vi "Mathematical interpolation.vi"(10 "Input data":dbl[][](array[numeric]), 11 "Method":i32(ring)=3 items=["nearest", "linear", "spline", "cubic Hermite", "Lagrange"]) -> (2 "Interpolated Data":dbl[][](array[numeric]), 3 "1D Interpolation Graph":cluster{"yi":dbl[], "ramp data":dbl[]}[](graph))   [LabVIEW 2017]
uses:
  <vilib>/Analysis/1siggen.llb/Ramp Pattern by Delta.vi
  <vilib>/gmath/NI_Gmath.lvlib
  <vilib>/Analysis/NI_AALBase.lvlib
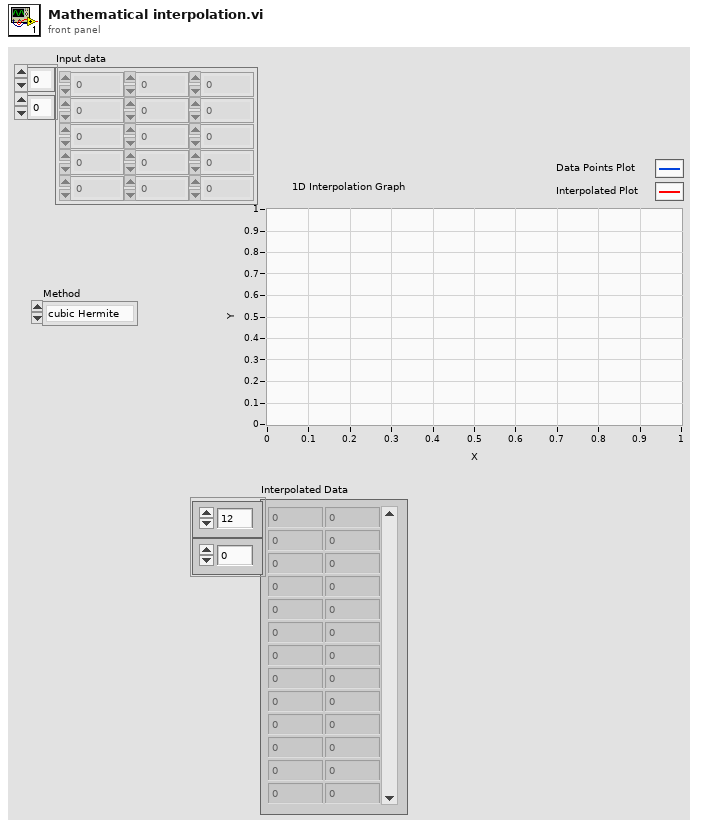
[diagram p1: front panel]
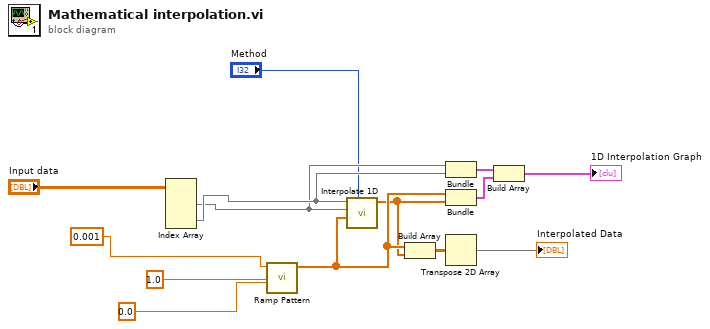
[diagram p0: block diagram]
diagram:
  n1 = Index Array(array="Input data") -> (element #1=w4:dbl[], element #2=w5:dbl[])  [unwired: 4 in]
  n2 = call-poly <vilib>:"Ramp Pattern.vi"("start"=0.0, "end"=1.0, "delta"=0.001) -> ("Ramp Pattern"=w8:dbl[])  [unwired: 6 in, 2 out]
  n3 = call <vilib>:"Interpolate 1D.vi"("method"="Method", "xi"=w8, "X"=w4, "Y"=w5) -> ("yi"=w7:dbl[])  [unwired: 5 in, 2 out]
  n4 = Build Array(w8, w7) -> (w6:dbl[][])
  n5 = Bundle("Input data"=w4, "Input data"=w5) -> (w3:cluster{"Input data":dbl[], "Input data":dbl[]})  [unwired: 1 in]
  n6 = Bundle("Ramp Pattern"=w8, "yi"=w7) -> (w2:cluster{"Ramp Pattern":dbl[], "yi":dbl[]})  [unwired: 1 in]
  n7 = Transpose 2D Array(2D array=w6) -> (transposed array=→"Interpolated Data":dbl[][])
  n8 = Build Array(w3, w2) -> (→"1D Interpolation Graph":cluster{"Ramp Pattern":dbl[], "yi":dbl[]}[])
